vi "Compute 1-Exp Gate Array.vi"(6 "A (1)":dbl=1.0, 8 "Error In":errorcluster, 9 "Gates Definitions":T3={"First Gate: t1"=0.0, "Gate Width: W"=0.0, "Gate Step: d"=0.0, "# Gates: G"=0.0, "Use Gate Center"=FALSE, "Frames/Image: F"=50, "Gates/Frame: L"=0, "Bits/Frame: q"=0, "Multiplicity: p"=0, "Gate Type"=enum."Square", "Gate Edge s"=4.0, "Gate Top Slope"=4.0, "Reversed Sawtooth?"=FALSE, "Computation"=FALSE, "User-defined Gate"={"X Array"=[], "Y Array"=[]}, "Tolerance"=50.0, "Integration"=enum."Item 0", "# Steps"=50.0, "Type of User-defined Function"=enum."Gate"}, 11 "Decay Definition":T1={"offset: t0"=0.0, "period: T"=0.0, "lifetime: tau"=0.0, "Incident Signal: I"=0.5, "Normalized Decays"=FALSE, "IRF Model"=enum."Dirac", "IRF Parameter 1"=0.0, "Poisson Signal"=FALSE}) -> (0 "Error Out":errorcluster, 1 "Gate Array":dbl[](array[numeric]), 3 "t Array":dbl[](array[numeric]))   [LabVIEW 2019]
uses:
  Gate Definitions.ctl
  Gate Type.ctl
  Graphs/XY Graph/XY Plot Data.ctl
  Decay Definiton.ctl
  IRF Model.ctl
panel:
  out "Cases (debug)":string[](array[string])
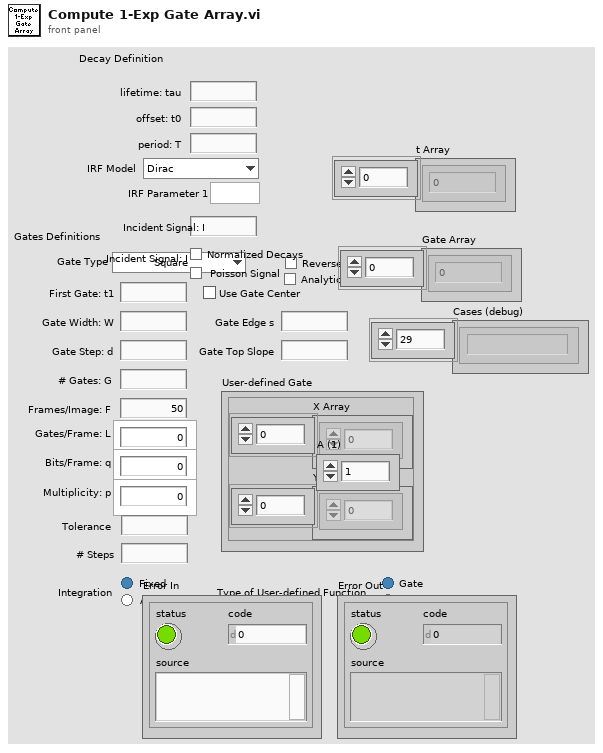
[diagram p1: front panel]
types:
  T1 = typedef "Decay Definiton.ctl" = cluster{"offset: t0":ext, "period: T":ext, "lifetime: tau":ext, "Incident Signal: I":ext, "Normalized Decays":bool, "IRF Model":T2, "IRF Parameter 1":ext, "Poisson Signal":bool}
  T2 = typedef "IRF Model.ctl" = enum16{"Dirac", "Exponential"}
  T3 = typedef "Gate Definitions.ctl" = cluster{"First Gate: t1":ext, "Gate Width: W":ext, "Gate Step: d":ext, "# Gates: G":ext, "Use Gate Center":bool, "Frames/Image: F":i32, "Gates/Frame: L":i32, "Bits/Frame: q":i32, "Multiplicity: p":i32, "Gate Type":T4, "Gate Edge s":ext, "Gate Top Slope":ext, "Reversed Sawtooth?":bool, "Computation":bool, "User-defined Gate":T5, "Tolerance":ext, "Integration":enum32{"Item 0", "Item 1"}, "# Steps":ext, "Type of User-defined Function":enum32{"Gate", "IRF"}}
  T4 = typedef "Gate Type.ctl" = enum16{"Square", "Finite Edge Square", "Finite Edge, Tilted Top Square", "Triangle", "Sawtooth", "User-defined"}
  T5 = typedef "XY Plot Data.ctl" = cluster{"X Array":dbl[], "Y Array":dbl[]}
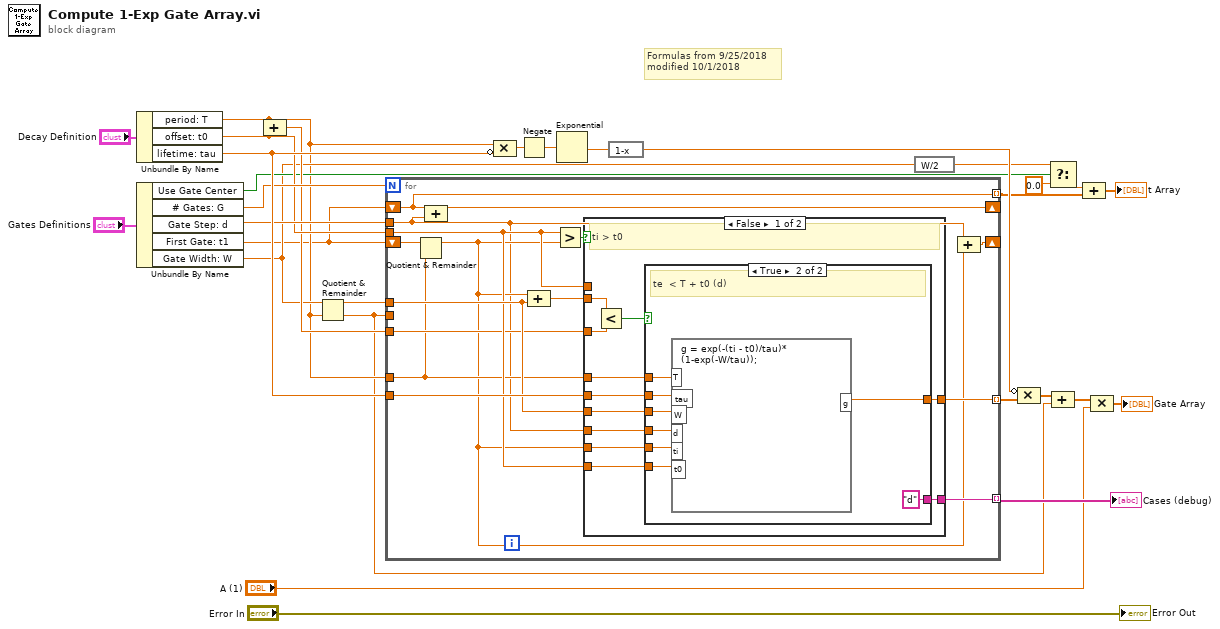
[diagram p0: block diagram]
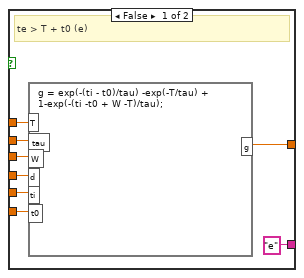
[diagram p2: hidden frame]
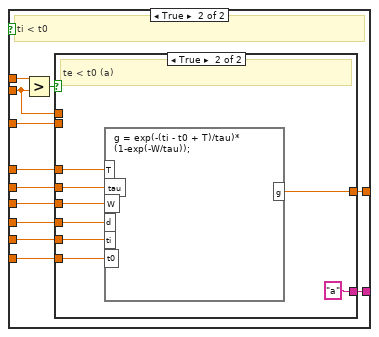
[diagram p3: hidden frame]
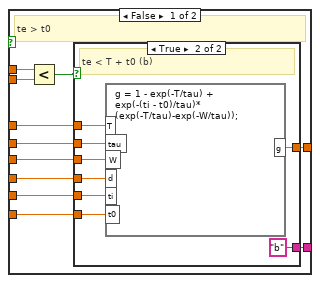
[diagram p4: hidden frame]
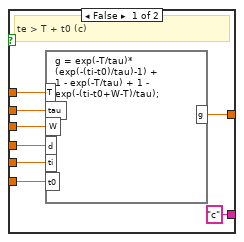
[diagram p5: hidden frame]
diagram:
  # "Formulas from 9/25/2018\nmodified 10/1/2018"
  n1 = Unbundle By Name("Decay Definition") -> ("period: T"=w7:ext, "offset: t0"=w17:ext, "lifetime: tau"=w25:ext)
  n2 = Unbundle By Name("Gates Definitions") -> ("Use Gate Center"=w13:bool, "# Gates: G"=w23:ext, "Gate Step: d"=w24:ext, "First Gate: t1"=w2:ext, "Gate Width: W"=w9:ext)
  n3 = Compound Arithmetic op=ADD(w7, w17) -> (w16:ext)
  n4 = Quotient & Remainder(x=w9, y=w7) -> (x-y*floor(x/y)=w8:ext, floor(x/y)=w5:ext)
  n5 = for {
    N: w23 -> [_]
    shift-right: [w44] -> _
    shift-left: w2 -> [w34]
    tunnel: w24 -> [w32]
    tunnel: w8 -> [w39]
    tunnel: w17 -> [w38]
    tunnel: w7 -> [w35]
    tunnel: [w41] -> w19 mode=indexing
    tunnel: w25 -> [w40]
    tunnel: w16 -> [w37]
    tunnel: [w36] -> w15 mode=indexing
    tunnel: w5 -> [_]
    shift-right: [w31] -> _
    shift-left: w2 -> [w30]
    tunnel: [w30] -> w1 mode=indexing
    n6 = Quotient & Remainder(x=w34, y=w35) -> (x-y*floor(x/y)=w33:ext)  [unwired: 1 out]
    n7 = Compound Arithmetic op=ADD(w30, w32) -> (w31:ext)
    n8 = Compound Arithmetic op=ADD(w33, w39) -> (w42:ext)
    n9 = Greater?(x=w38, y=w33) -> (0:w43:bool)
    n10 = case shown="False" w43 {
      tunnel: w42 -> [w55 w81]
      tunnel: w38 -> [_ w83]
      tunnel: w35 -> [w48 w74]
      tunnel: [w47 w80] -> w41
      tunnel: w40 -> [w49 w79]
      tunnel: w39 -> [w50 w78]
      tunnel: w32 -> [w51 w77]
      tunnel: w33 -> [w52 w76]
      tunnel: w38 -> [w53 w75]
      tunnel: w37 -> [w45 w73]
      tunnel: [w46 w72] -> w36
      frame False {
        # "ti > t0"
        n11 = Less?(x=w55, y=w45) -> (x < y?=w54:bool)
        n12 = case shown="True" w54 {
          tunnel: w53 -> [w58 w71]
          tunnel: w52 -> [w59 w70]
          tunnel: w51 -> [w60 w69]
          tunnel: w50 -> [w61 w68]
          tunnel: w49 -> [w62 w67]
          tunnel: w48 -> [w63 w66]
          tunnel: [w57 w65] -> w47
          tunnel: ["e" "d"] -> w46
          frame False {
            # "te > T + t0 (e)"
            n13 = formula code="g = exp(-(ti - t0)/tau) -exp(-T/tau) +\n1-exp(-(ti -t0 + W -T)/tau);"("T"=w63, "ti"=w59, "tau"=w62, "W"=w61, "d"=w60, "t0"=w58) -> ("g"=w57:dbl)
          }
          frame True {
            # "te  < T + t0 (d)"
            n14 = formula code="g = exp(-(ti - t0)/tau)*\n(1-exp(-W/tau));"("T"=w66, "ti"=w70, "tau"=w67, "W"=w68, "d"=w69, "t0"=w71) -> ("g"=w65:dbl)
          }
        }
      }
      frame True {
        # "ti < t0"
        n15 = Greater?(x=w83, y=w81) -> (0:w82:bool)
        n16 = case shown="True" w82 {
          tunnel: w81 -> [w87 _]
          tunnel: w74 -> [w86 w112]
          tunnel: [w93 w113] -> w80
          tunnel: w79 -> [w92 w118]
          tunnel: w78 -> [w91 w117]
          tunnel: w77 -> [w90 w116]
          tunnel: w76 -> [w89 w115]
          tunnel: w75 -> [w88 w114]
          tunnel: w73 -> [w85 _]
          tunnel: [w84 "a"] -> w72
          frame False {
            # "te > t0"
            n17 = Less?(x=w87, y=w85) -> (x < y?=w94:bool)
            n18 = case shown="True" w94 {
              tunnel: [w102 w104] -> w93
              tunnel: w86 -> [w101 w110]
              tunnel: w92 -> [w100 w109]
              tunnel: w91 -> [w99 w108]
              tunnel: w90 -> [w98 w107]
              tunnel: w89 -> [w97 w106]
              tunnel: w88 -> [w96 w105]
              tunnel: ["c" "b"] -> w84
              frame False {
                # "te > T + t0 (c)"
                n19 = formula code="g = exp(-T/tau)*\n(exp(-(ti-t0)/tau)-1) +\n1 - exp(-T/tau) + 1 - \nexp(-(ti-t0+W-T)/tau);"("T"=w101, "ti"=w97, "tau"=w100, "W"=w99, "d"=w98, "t0"=w96) -> ("g"=w102:dbl)
              }
              frame True {
                # "te < T + t0 (b)"
                n20 = formula code="g = 1 - exp(-T/tau) + \nexp(-(ti - t0)/tau)*\n(exp(-T/tau)-exp(-W/tau));"("T"=w110, "ti"=w106, "tau"=w109, "W"=w108, "d"=w107, "t0"=w105) -> ("g"=w104:dbl)
              }
            }
          }
          frame True {
            # "te < t0 (a)"
            n21 = formula code="g = exp(-(ti - t0 + T)/tau)*\n(1-exp(-W/tau));"("T"=w112, "ti"=w115, "tau"=w118, "W"=w117, "d"=w116, "t0"=w114) -> ("g"=w113:dbl)
          }
        }
      }
    }
    n22 = Compound Arithmetic op=ADD(w32, w33) -> (w44:ext)
  }
  "Cases (debug)" <- w15
  n23 = Compound Arithmetic op=MULTIPLY(w7, invert w25) -> (w26:ext)
  n24 = Negate(x=w26) -> (-x=w27:ext)
  n25 = Exponential(1:w27) -> (0:w28:ext)
  n26 = expression code="1-x"(w28) -> (w29:ext)
  n27 = expression code="W/2"(w9) -> (w10:ext)
  n28 = Compound Arithmetic op=MULTIPLY(invert w29, w19) -> (w20:ext[])
  n29 = Select(t=w10, s=w13, f=0.0 ("t")) -> (s? t:f=w12:ext)
  n30 = Compound Arithmetic op=ADD(w20, w5) -> (w6:ext[])
  n31 = Compound Arithmetic op=ADD(w12, w1) -> (→"t Array":ext[])
  n32 = Compound Arithmetic op=MULTIPLY(w6, "A (1)") -> (→"Gate Array":ext[])
  "Error Out" <- "Error In"
